vi "Get Return - Pythonic.vi"(7 "Function Name":string, 8 "Error In":errorcluster, 11 "OPI Ref":refnum<data-value>) -> (0 "Error Out":errorcluster, 1 "Pythonic Return Value":string, 3 "OPI Ref":refnum<data-value>)   [LabVIEW 2012, in "OPI.lvclass"]
doc: "Get return value from previously made function call, specified by Function Name. The returned value will be provided in pythonic string format. Use Converter method to translate it into LabVIEW data.\n\n<b>Important</b> - use this method to translate pythonic tuples and dictionaries.\n\nProviding data like this makes the OPI as flexible as possible, allowing work with any python type that flattens to string."
uses:
  OPI.lvclass
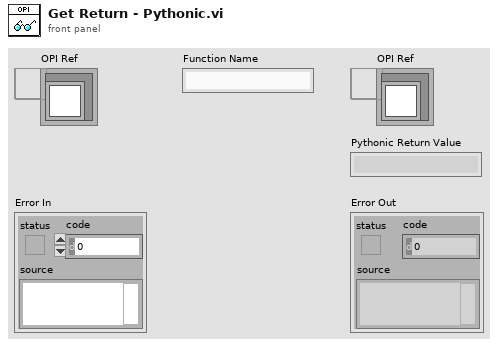
[diagram p1: front panel]
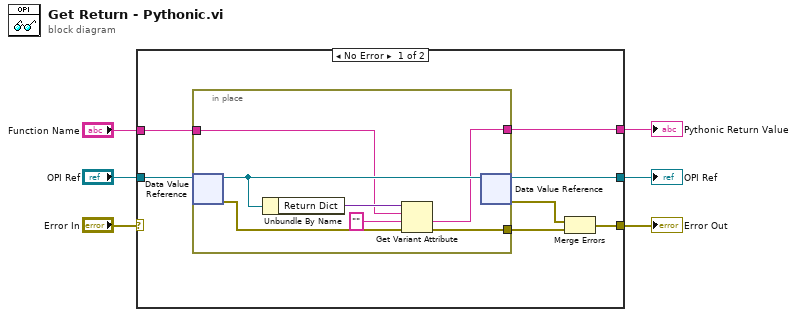
[diagram p0: block diagram]
diagram:
  n1 = case shown="No Error" "Error In" {
    selector: "Error In" -> [_ w22]
    tunnel: "OPI Ref" -> [w13 w21]
    tunnel: [w12 w21] -> w5
    tunnel: "Function Name" -> [w11 _]
    tunnel: [w10 _] -> w3
    tunnel: [w7 w22] -> w1
    frame No Error {
      n2 = in-place {
        in-place-border: w11 -> [w18]
        in-place-border: [w17] -> w10
        in-place-border: [w15] -> w8
        n3 = in-place-dvr #1(w13) -> (w19:refnum<class "OPI.lvclass">, w16:errorcluster)
        n4 = Unbundle By Name(w19) -> ("Return Dict"=w20:variant)
        n5 = Get Variant Attribute(Variant=w20, name=w18, default value (empty Variant)="", error in=w16) -> (value=w17:string, error out=w15:errorcluster)  [unwired: 2 out]
        n6 = in-place-dvr #1(w19) -> (w12:refnum<data-value>, w9:errorcluster)
      }
      n7 = Merge Errors(w9, w8) -> (w7:errorcluster)
    }
    frame Error {
    }
  }
  "Error Out" <- w1
  "OPI Ref" <- w5
  "Pythonic Return Value" <- w3
